vi "Class creation memory test.vi"() -> ()   [LabVIEW 2022 SP3]
uses:
  Public/Classes/IInstanceBuilder/IInstanceBuilder.lvclass
panel:
  out "Exec. time [s]":dbl
  out "error out":errorcluster
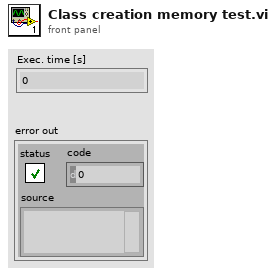
[diagram p1: front panel]
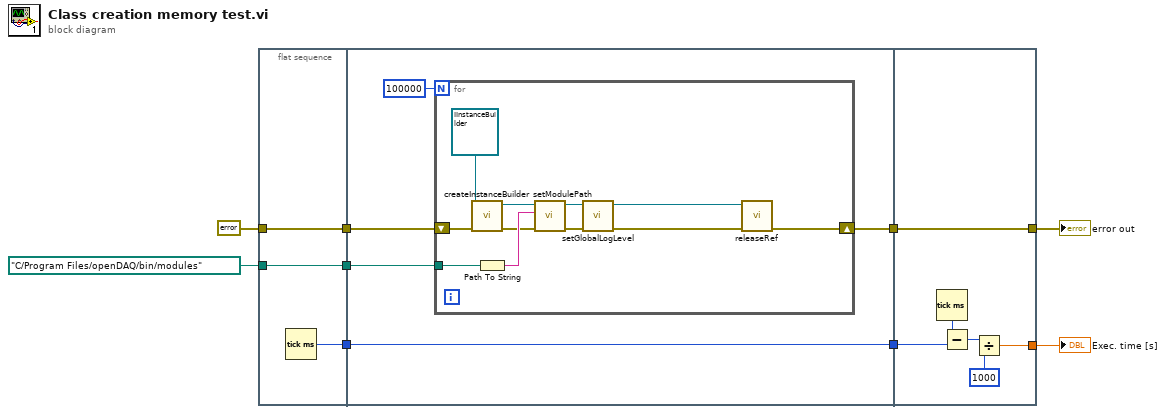
[diagram p0: block diagram]
diagram:
  n1 = flat-sequence {
    tunnel: errorcluster {"status"=FALSE, "code"=0, "source"=""} ("error in (no error)") -> [w11]
    tunnel: path "C:/Program Files/openDAQ/bin/modules" -> [w12]
    tunnel: [w12] -> w6
    tunnel: [w11] -> w5
    tunnel: [w10] -> w1
    tunnel: w6 -> [w17]
    tunnel: w5 -> [w16]
    tunnel: [w15] -> w4
    tunnel: [w13] -> w2
    tunnel: w1 -> [w13]
    tunnel: [w34] -> w7
    tunnel: w4 -> [w34]
    tunnel: [w31] -> w3
    tunnel: w2 -> [w30]
    frame #0 {
      n2 = Tick Count (ms)() -> (millisecond timer value=w10:u32)
    }
    frame #1 {
      n3 = for {
        N: 100000 -> [_]
        tunnel: w17 -> [w28]
        shift-right: [w22] -> w15
        shift-left: w16 -> [w23]
        n4 = call "createInstanceBuilder.vi"("error in (no error)"=w23, "IInstanceBuilder in"=refnum<class "IInstanceBuilder.lvclass"> refnum ("openDAQ.lvlib:IInstanceBuilder.lvclass")) -> ("error out"=w24:errorcluster, "IInstanceBuilder out"=w26:refnum<class "IInstanceBuilder.lvclass">)  [unwired: 8 in]
        n5 = Path To String(path=w28) -> (string=w25:string)
        n6 = call "setModulePath.vi"("error in (no error)"=w24, "modulePathStr"=w25, "IInstanceBuilder in"=w26) -> ("error out"=w19:errorcluster, "IInstanceBuilder out"=w21:refnum<class "IInstanceBuilder.lvclass">)  [unwired: 7 in]
        n7 = call "setGlobalLogLevel.vi"("error in (no error)"=w19, "IInstanceBuilder in"=w21) -> ("error out"=w18:errorcluster, "IInstanceBuilder out"=w20:refnum<class "IInstanceBuilder.lvclass">)  [unwired: 8 in]
        n8 = call-dynamic "releaseRef.vi"("error in (no error)"=w18, "IBaseObject in"=w20) -> ("error out"=w22:errorcluster)  [unwired: 9 in]
      }
    }
    frame #2 {
      n9 = Tick Count (ms)() -> (millisecond timer value=w29:u32)
      n10 = Subtract(x=w29, y=w30) -> (x-y=w33:u32)
      n11 = Divide(x=w33, y=u32 1000) -> (x/y=w31:dbl)
    }
  }
  "error out" <- w7
  "Exec. time [s]" <- w3
